vi "createMissionWaypoints.vi"(8 "error in (no error)":errorcluster, 11 "StationKeeping in":refnum<class "StationKeeping.lvclass">) -> (0 "error out":errorcluster, 3 "StationKeeping out":refnum<class "StationKeeping.lvclass">)   [LabVIEW 2011, in "StationKeeping.lvclass"]
uses:
  StationKeeping.lvclass
  StationKeeping.lvclass/StationKeeping.ctl
  2 Globals/2 Global.vi
  Waypoint/Waypoint.lvclass
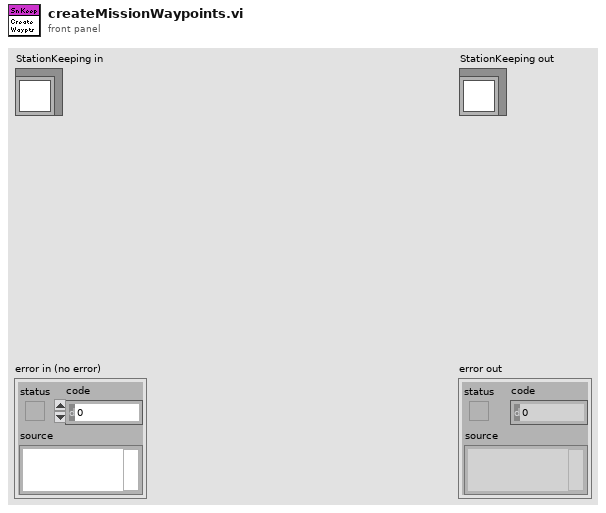
[diagram p1: front panel]
types:
  T1 = typedef "UTM Location.ctl" = cluster{"UTM Zone":dbl, "Hemisphere":enum16{"North", "South"}, "East":dbl, "North":dbl}
  T2 = typedef "UTM Circle.ctl" = cluster{"UTM Zone":dbl, "Hemisphere":enum16{"North", "South"}, "East":dbl, "North":dbl, "Radius":dbl}
  T3 = typedef "Waypoints List.ctl" = refnum<class "Waypoint.lvclass">[]
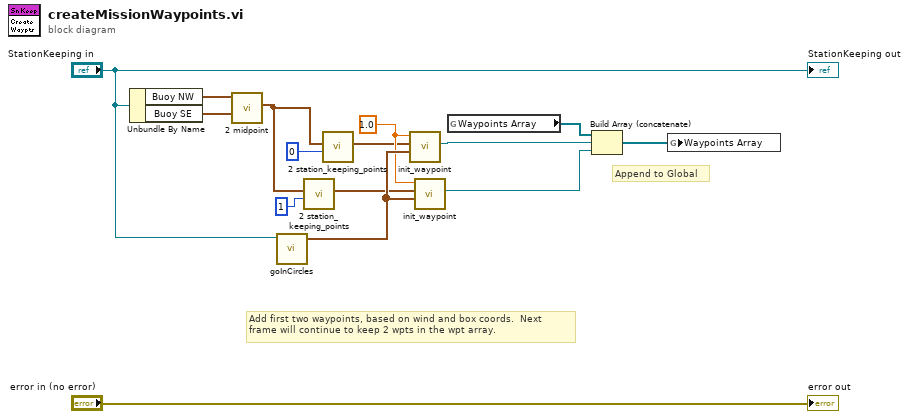
[diagram p0: block diagram]
diagram:
  w11 = 1.0 ("Tolerance (meters?)")
  # "Append to Global"
  # "Add first two waypoints, based on wind and box coords.  Next\nframe will continue to keep 2 wpts in the wpt array."
  n1 = Unbundle By Name("StationKeeping in") -> ("Buoy NW"=w4:T1, "Buoy SE"=w3:T1)
  n2 = call "2 midpoint.vi"("UTM 2"=w3, "UTM 1"=w4) -> ("Midpoint"=w8:T1)  [unwired: 8 in, 1 out]
  n3 = call "goInCircles.vi"("StationKeeping in"="StationKeeping in") -> ("No Sail Circles"=w12:T2[])  [unwired: 8 in, 2 out]
  n4 = call "2 station_keeping_points.vi"("Which Point?"=1, "Midpoint"=w8) -> ("Waypoint"=w10:T1)  [unwired: 9 in]
  n5 = call "2 station_keeping_points.vi"("Which Point?"=0, "Midpoint"=w8) -> ("Waypoint"=w9:T1)  [unwired: 9 in]
  n6 = call "init_waypoint.vi"("No Sail Circles"=w12, "Coords"=w9, "Tolerance (m)"=w11) -> ("Waypoint Out"=w14:refnum<class "Waypoint.lvclass">)  [unwired: 8 in]
  n7 = call "init_waypoint.vi"("No Sail Circles"=w12, "Coords"=w10, "Tolerance (m)"=w11) -> ("Waypoint Out"=w13:refnum<class "Waypoint.lvclass">)  [unwired: 8 in]
  n8 = global read "2 Global.vi" "Waypoints Array"() -> (w15:T3)
  n9 = Build Array (concatenate)(w15, w14, w13) -> (w5:T3)
  n10 = global write "2 Global.vi" "Waypoints Array"(w5) -> ()
  "error out" <- "error in (no error)"
  "StationKeeping out" <- "StationKeeping in"
